vi "判断表格的存档日期是否要更新.vi"(9 "各Sheet名称数组":string[](array[string]), 10 "ModelEditInfo输入":T1={"AllModelFold"=path "", "AllModelNamePath"=path "", "所有零件型号"=[], "当前零件型号"="", "所有建立零件信息"=[], "当前零件序号"=0, "当前产品信息"={"产品型号"="J016-9STWH-A插头", "二维码拍照"=0, "Mark点拍照"=0}}, 11 "已经存在路径":path) -> (0 "错误out":errorcluster caption="错误常量", 3 "当天存数据路径":path)   [LabVIEW 2014]
uses:
  ModelEditSubVIs/ModeEditeControl.ctl
  ModelEditSubVIs/ModelInfo.ctl
  Global.vi
panel:
  out "x-y":u32
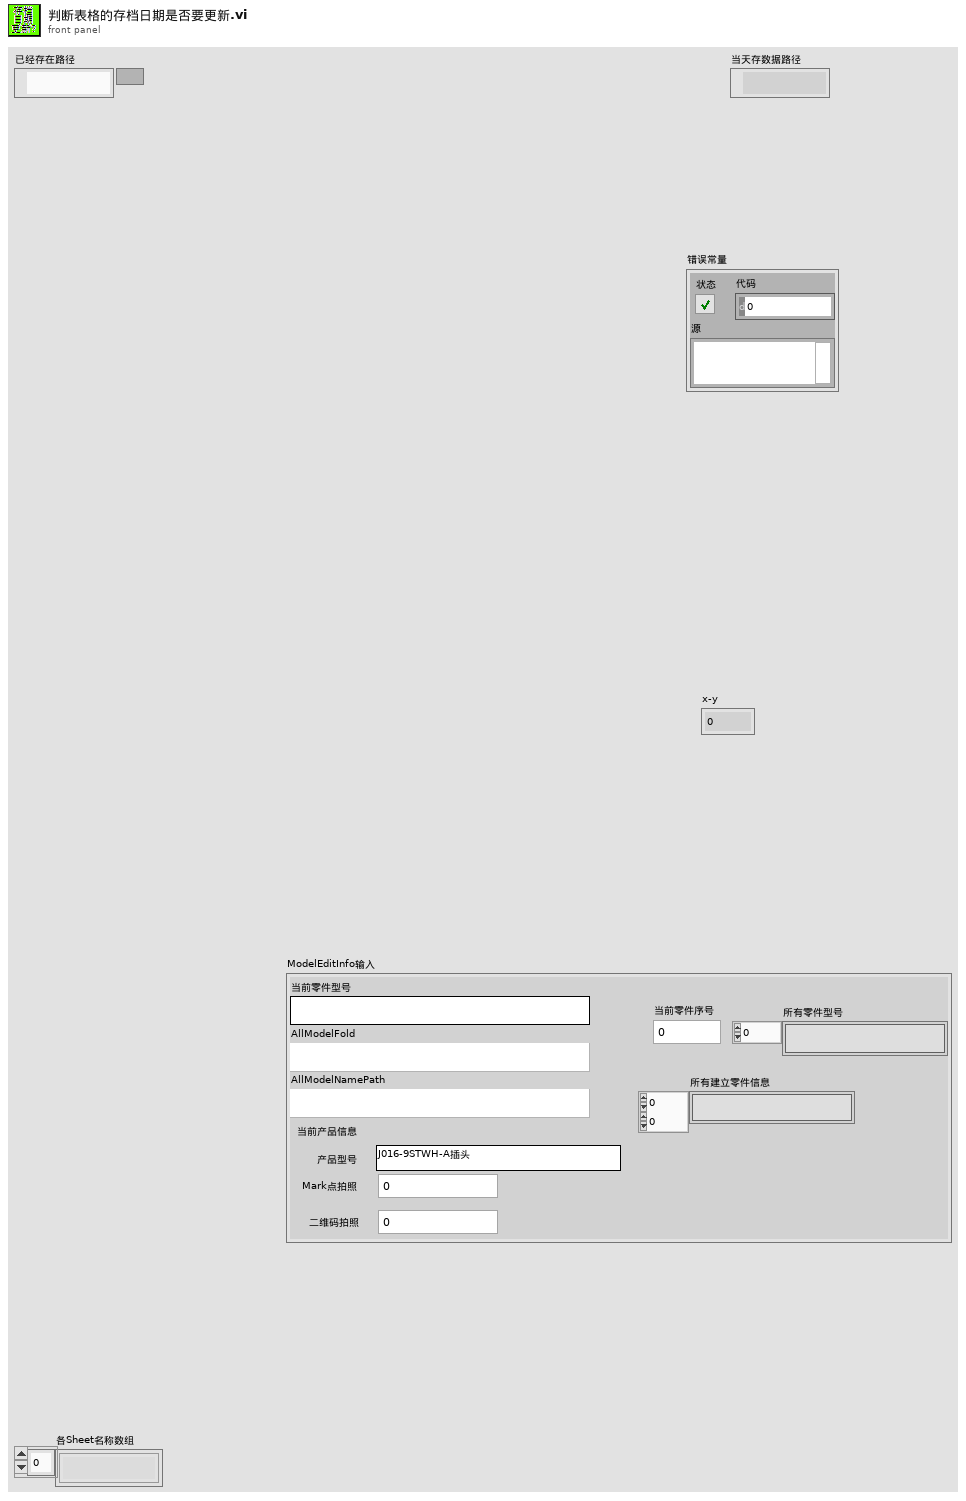
[diagram p1: front panel]
types:
  T1 = typedef "ModeEditeControl.ctl" = cluster{"AllModelFold":path, "AllModelNamePath":path, "所有零件型号":string[], "当前零件型号":string, "所有建立零件信息":string[][], "当前零件序号":i32, "当前产品信息":T2}
  T2 = typedef "ModelInfo.ctl" = cluster{"产品型号":string, "二维码拍照":u32, "Mark点拍照":u32}
  T3 = typedef "控件-Excel读写选项.ctl" = enum16{"打开表格", "新增sheet", "读取sheet指定位置数据", "读取sheet整个数据", "写入sheet整个数据", "写表头", "数据存到本机", "表格是否开启状态", "关闭表格"}
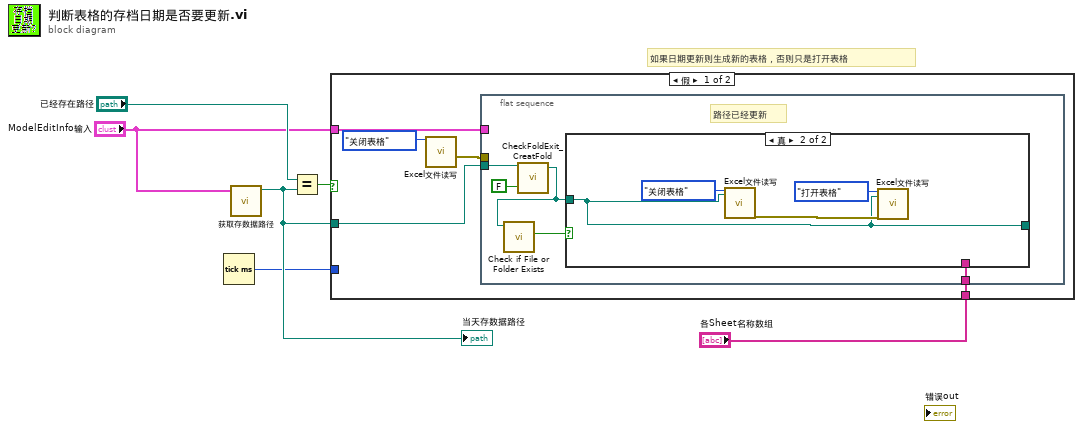
[diagram p0: block diagram]
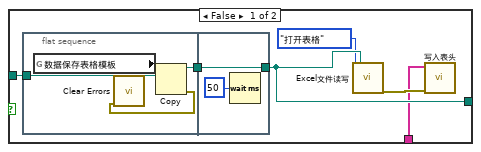
[diagram p2: hidden frame]
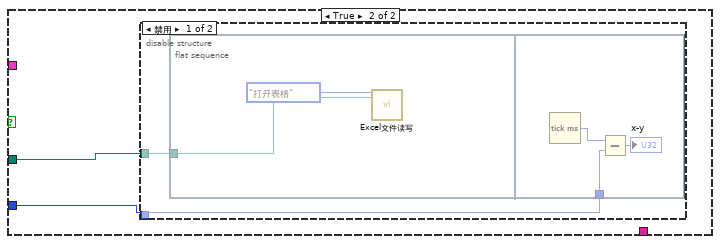
[diagram p3: hidden frame]
diagram:
  # "如果日期更新则生成新的表格，否则只是打开表格"
  n1 = Tick Count (ms)() -> (millisecond timer value=w2:u32)
  n2 = call "获取存数据路径.vi"("ModelEditInfo"="ModelEditInfo输入") -> ("当天存数据路径"=w5:path)  [unwired: 10 in]
  "当天存数据路径" <- w5
  n3 = Equal?(x="已经存在路径", y=w5) -> (x = y?=w3:bool)
  n4 = case shown="假" w3 {
    tunnel: w5 -> [w11 w34]
    tunnel: "ModelEditInfo输入" -> [w10 _]
    tunnel: "各Sheet名称数组" -> [w9 _]
    tunnel: w2 -> [_ w33]
    frame False {
      n5 = call "Excel文件读写.vi"("选项"=控件-Excel读写选项."关闭表格") -> ("error out"=w7:errorcluster)  [unwired: 16 in, 2 out]
      n6 = flat-sequence {
        tunnel: w11 -> [w13]
        tunnel: w10 -> [_]
        tunnel: w9 -> [w12]
        tunnel: w7 -> [_]
        frame #0 {
          # "路径已经更新"
          n7 = call "CheckFoldExit_CreatFold.vi"("path in"=w13, "FoldOrFile¡H"=FALSE) -> ("File out"=w16:path)  [unwired: 2 out]
          n8 = call <vilib>:"Check if File or Folder Exists.vi"("path"=w16) -> ("file or folder exists?"=w15:bool)  [unwired: 1 in, 9 out]
          n9 = case shown="真" w15 {
            tunnel: w16 -> [w21 w31]
            tunnel: [w20 w31] -> _
            tunnel: w12 -> [w17 _]
            frame False {
              n10 = flat-sequence {
                tunnel: w21 -> [w26]
                tunnel: [w24] -> w22
                tunnel: w22 -> [w27]
                tunnel: [w27] -> w20
                frame #0 {
                  n11 = global read "Global.vi" "数据保存表格模板"() -> (w25:path)
                  n12 = Copy(10:w26, 11:w25) -> (0:w23:errorcluster, 3:w24:path)  [unwired: 3 in, 1 out]
                  n13 = call <vilib>:"Clear Errors.vi"("error in (no error)"=w23) -> ()  [unwired: 5 in, 2 out]
                }
                frame #1 {
                  n14 = Wait (ms)(milliseconds to wait=u32 50 ("等待时间（毫秒）")) -> ()  [unwired: 1 out]
                }
              }
              n15 = call "Excel文件读写.vi"("选项"=控件-Excel读写选项."打开表格", "Path"=w20) -> ("error out"=w18:errorcluster)  [unwired: 15 in, 2 out]
              n16 = call "写入表头.vi"("错误in"=w18, "各sheet名称数组"=w17) -> ()  [unwired: 10 in]
            }
            frame True {
              n17 = call "Excel文件读写.vi"("选项"=控件-Excel读写选项."关闭表格", "Path"=w31) -> ("error out"=w32:errorcluster)  [unwired: 15 in, 2 out]
              n18 = call "Excel文件读写.vi"("选项"=控件-Excel读写选项."打开表格", "error in"=w32, "Path"=w31) -> ()  [unwired: 14 in, 3 out]
            }
          }
        }
      }
    }
    frame True {
      n19 = disable-structure shown="禁用" {
        disable-tunnel: w34 -> [w36 _]
        disable-tunnel: w33 -> [w35 _]
        frame Disabled {
          n20 = flat-sequence {
            tunnel: w36 -> [w37]
            tunnel: w35 -> [w40]
            frame #0 {
              n21 = call "Excel文件读写.vi"("选项"=控件-Excel读写选项."打开表格", "sheet name"=w37) -> ()  [unwired: 15 in, 3 out]
            }
            frame #1 {
              n22 = Tick Count (ms)() -> (millisecond timer value=w41:u32)
              n23 = Subtract(x=w41, y=w40) -> (x-y=→"x-y":u32)
            }
          }
        }
        frame Enabled {
        }
      }
    }
  }
